vi "Generate_AO_Waveforms.vi"(8 "error in (no error)":errorcluster, 9 "sampling info":cluster{"Fs":dbl, "#s":dbl}={"Fs"=1000.0, "#s"=1000.0} {"Fs" format="%.2p"}, 10 "reset signal":bool, 11 "output config":T1(array[cluster])=[{"A (V)"=1.0, "DC (V)"=0.0, "f (Hz)"=1.0, "phi (deg)"=0.0, "signal type"=enum."Sine Wave"}, {"A (V)"=2.0, "DC (V)"=0.0, "f (Hz)"=2.0, "phi (deg)"=0.0, "signal type"=enum."Sine Wave"}, {"A (V)"=3.0, "DC (V)"=0.0, "f (Hz)"=3.0, "phi (deg)"=0.0, "signal type"=enum."Sine Wave"}, {"A (V)"=4.0, "DC (V)"=0.0, "f (Hz)"=4.0, "phi (deg)"=0.0, "signal type"=enum."Sine Wave"}, {"A (V)"=5.0, "DC (V)"=0.0, "f (Hz)"=5.0, "phi (deg)"=0.0, "signal type"=enum."Sine Wave"}, {"A (V)"=6.0, "DC (V)"=0.0, "f (Hz)"=6.0, "phi (deg)"=0.0, "signal type"=enum."Sine Wave"}, {"A (V)"=7.0, "DC (V)"=0.0, "f (Hz)"=7.0, "phi (deg)"=0.0, "signal type"=enum."Sine Wave"}]) -> (0 "error out":errorcluster, 2 "AO Array":waveform(dbl)[](array[waveform]))   [LabVIEW 2020, in "DAQ_Manager.lvclass"]
uses:
  DAQ_Manager.lvclass
  <vilib>/measure/NI_MABase.lvlib
panel:
  out "Numeric":i32
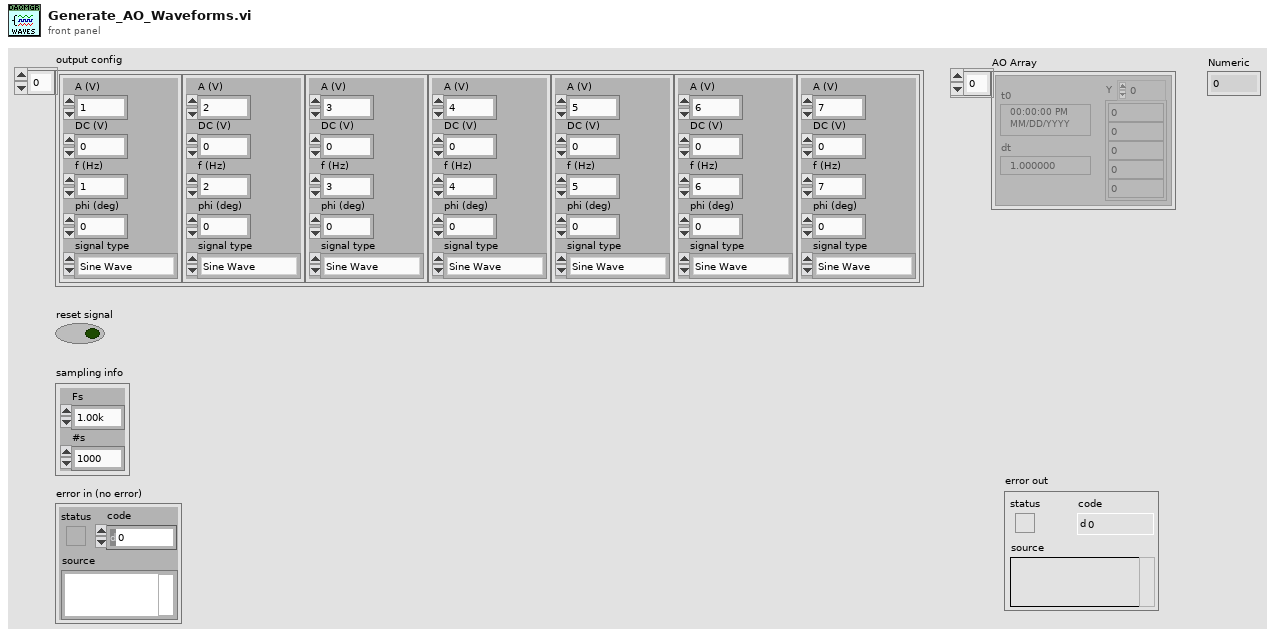
[diagram p1: front panel]
types:
  T1 = cluster{"A (V)":dbl, "DC (V)":dbl, "f (Hz)":dbl, "phi (deg)":dbl, "signal type":enum16{"Sine Wave", "Triangle Wave", "Square Wave", "Sawtooth Wave"}}[]
  T2 = enum16{"Sine Wave", "Triangle Wave", "Square Wave", "Sawtooth Wave"}
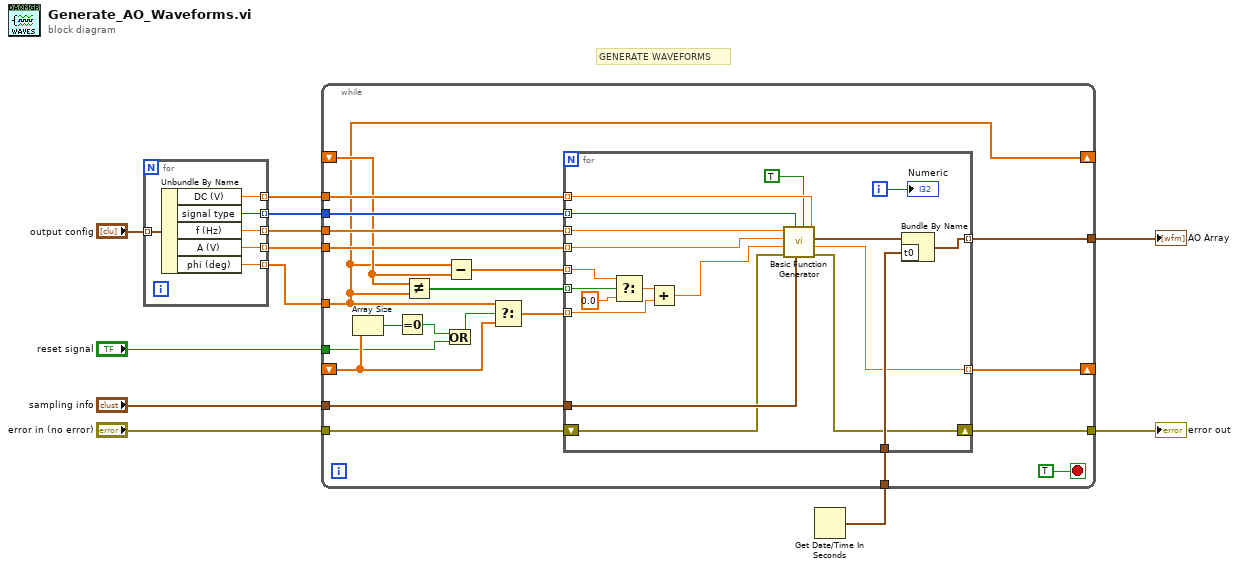
[diagram p0: block diagram]
diagram:
  # "GENERATE WAVEFORMS"
  n1 = for {
    tunnel: "output config" -> [w18] mode=indexing
    tunnel: [w17] -> w8 mode=indexing
    tunnel: [w16] -> w7 mode=indexing
    tunnel: [w15] -> w6 mode=indexing
    tunnel: [w14] -> w5 mode=indexing
    tunnel: [w13] -> w4 mode=indexing
    n2 = Unbundle By Name(w18) -> ("DC (V)"=w17:dbl, "signal type"=w16:T2, "f (Hz)"=w15:dbl, "A (V)"=w14:dbl, "phi (deg)"=w13:dbl)
  }
  n3 = Get Date/Time In Seconds() -> (seconds since 1Jan1904=w10:timestamp)
  n4 = while {
    tunnel: w7 -> [w39]
    tunnel: w8 -> [w38]
    tunnel: "sampling info" -> [w21]
    tunnel: [w37] -> w1
    tunnel: w5 -> [w36]
    tunnel: w4 -> [w27]
    tunnel: w6 -> [w35]
    shift-right: [w27] -> _
    shift-left: _ -> [w32]
    shift-right: [w30] -> _
    shift-left: _ -> [w24]
    tunnel: w10 -> [w29]
    tunnel: "reset signal" -> [w22]
    tunnel: "error in (no error)" -> [w20]
    tunnel: [w19] -> w2
    stop <- TRUE stop-if-true
    n5 = Array Size(array=w24) -> (size(s)=w28:i32)
    n6 = Equal To 0?(x=w28) -> (x = 0?=w23:bool)
    n7 = Not Equal?(x=w32, y=w27) -> (x != y?=w33:bool[])
    n8 = Or(x=w23, y=w22) -> (x .or. y?=w26:bool)
    n9 = Subtract(x=w27, y=w32) -> (x-y=w31:dbl[])
    n10 = Select(t=w27, s=w26, f=w24) -> (s? t:f=w25:dbl[])
    n11 = for {
      tunnel: w39 -> [w58] mode=indexing
      tunnel: w35 -> [w57] mode=indexing
      tunnel: w36 -> [w56] mode=indexing
      tunnel: w38 -> [w55] mode=indexing
      tunnel: [w46] -> w37 mode=indexing
      tunnel: w21 -> [w41]
      tunnel: w33 -> [w50] mode=indexing
      tunnel: w31 -> [w52] mode=indexing
      tunnel: [w44] -> w30 mode=indexing
      tunnel: w25 -> [w43] mode=indexing
      tunnel: w29 -> [w49]
      shift-right: [w45] -> w19
      shift-left: w20 -> [w40]
      i -> [w48]
      n12 = Select(t=w52, s=w50, f=0.0) -> (s? t:f=w53:dbl)
      n13 = Add(x=w53, y=w43) -> (x+y=w42:dbl)
      n14 = call <vilib>:"Basic Function Generator.vi"("offset"=w55, "reset signal"=TRUE, "sampling info"=w41, "signal type"=w58, "error in (no error)"=w40, "phase"=w42, "amplitude"=w56, "frequency"=w57) -> ("error out"=w45:errorcluster, "phase out"=w44:dbl, "signal out"=w54:waveform(dbl))  [unwired: 1 in]
      n15 = Bundle By Name(cluster=w54, "t0"=w49) -> (w46:waveform(dbl))
      "Numeric" <- w48
    }
  }
  "AO Array" <- w1
  "error out" <- w2
